vi "Save.vi"(8 "error in (no error)":errorcluster, 10 "Resampling Array":i32[](array[numeric]), 11 "DAQ Class in":refnum<class "DAQ Class.lvclass">) -> (0 "error out":errorcluster, 3 "DAQ Class out":refnum<class "DAQ Class.lvclass">)   [LabVIEW 2014, in "DAQ Class.lvclass"]
uses:
  DAQ Class.lvclass
  DAQ Class.lvclass/DAQ Class.ctl
  <vilib>/Utility/config.llb/Write Key (Double).vi
  <vilib>/Utility/config.llb/Write Key (I32).vi
  <vilib>/Utility/config.llb/Write Key (U32).vi
  <vilib>/Utility/config.llb/NI_LVConfig.lvlib
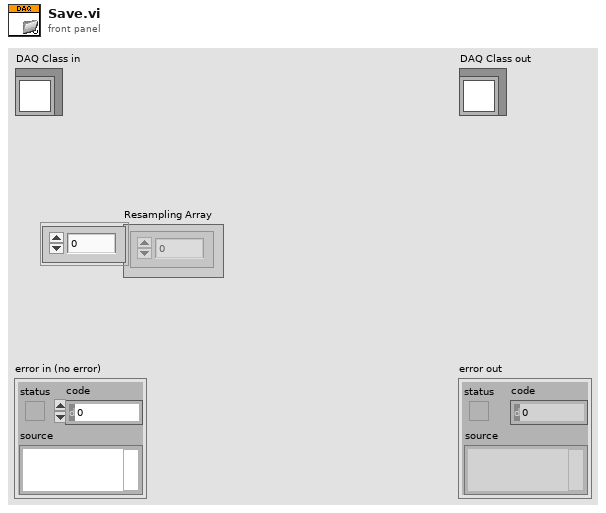
[diagram p1: front panel]
types:
  T1 = typedef "DAQ Class.lvclass/DAQ Parameters.ctl" = cluster{"Points Per A-Scan":u32, "A-Scans Per B-Scan":u32, "Number of B-Scans":u32, "A-Scans Per Transfer":u32, "Trigger Voltage":sgl, "Trigger Source":T2, "Trigger Slope":T3, "Channel":T4, "Clock":T5, "Bits per Sample":dbl, "Range":dbl}
  T2 = typedef "DAQ Class.lvclass/Trigger Source.ctl" = enum16{"External", "Channel A", "Channel B"}
  T3 = typedef "DAQ Class.lvclass/Trigger Slope.ctl" = enum16{"Rising", "Falling"}
  T4 = typedef "OCT DAQ Channel Data Type.ctl" = enum16{"Channel 1", "Channel 2", "Channel 1 and 2"}
  T5 = typedef "DAQ Class.lvclass/Clock Control.ctl" = enum16{"Internal Clock", "External Clock"}
  T6 = typedef "NI_LVConfig.lvlib/Config Data RefNum.ctl" = refnum<k1>
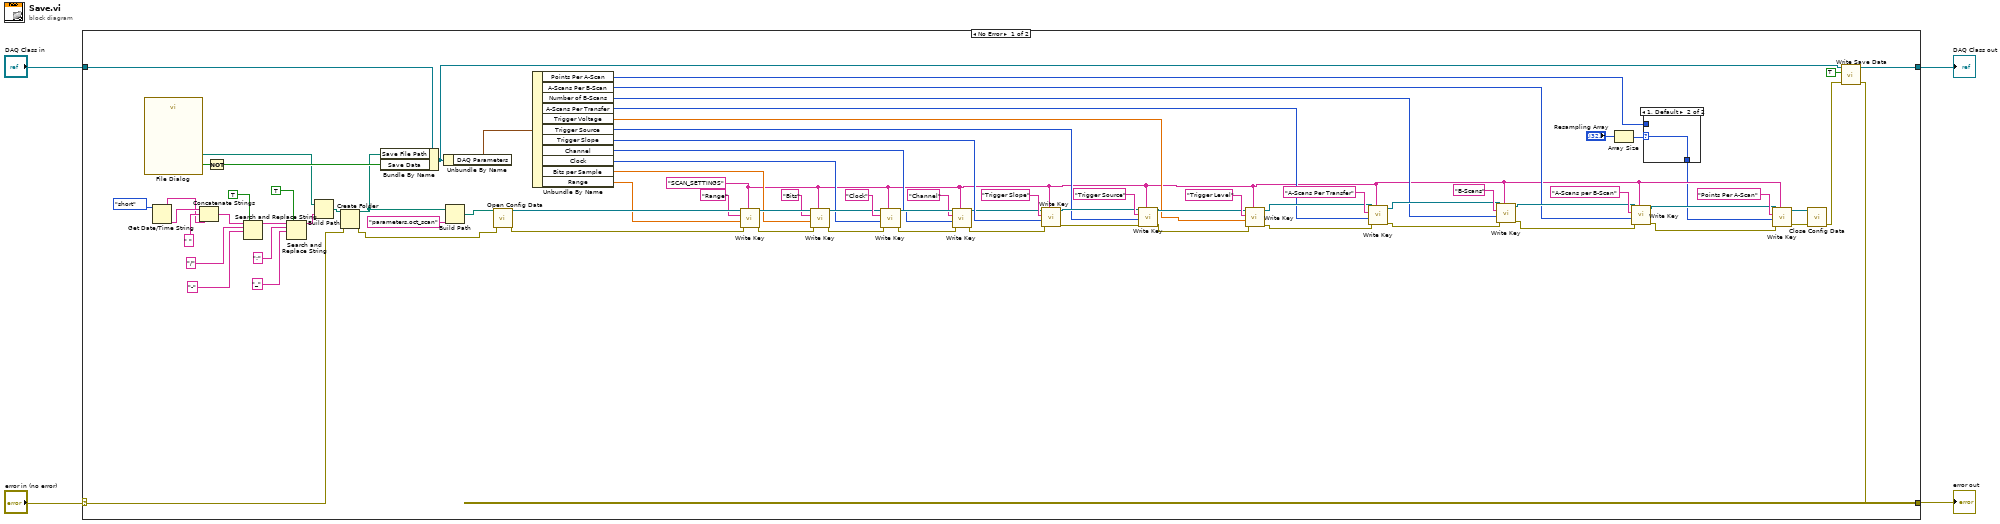
[diagram p0: block diagram]
diagram:
  n1 = case shown="No Error" "error in (no error)" {
    selector: "error in (no error)" -> [w66 w87]
    tunnel: [w8 w87] -> w3
    tunnel: [w7 w86] -> w1
    tunnel: "DAQ Class in" -> [w56 w86]
    frame No Error {
      w17 = "SCAN_SETTINGS" ("section")
      n2 = call "File Dialog"() -> ("selected path"=w77:path, "cancelled"=w83:bool)  [unwired: 12 in, 2 out]
      n3 = Get Date/Time String(date format (0)=enum16{"short", "long", "abbreviated"}."short") -> (date string=w79:string, time string=w80:string)  [unwired: 2 in]
      n4 = Concatenate Strings(w80, " " ("string"), w79) -> (w75:string)
      n5 = Not(x=w83) -> (.not. x?=w82:bool)
      n6 = Search and Replace String(replace all?=TRUE ("replace all? (F)"), input string=w75, search string="/", replace string="-" ("search string")) -> (result string=w72:string)  [unwired: 4 in, 3 out]
      n7 = Search and Replace String(replace all?=TRUE ("replace all? (F)"), input string=w72, search string=":", replace string="_" ("search string")) -> (result string=w71:string)  [unwired: 4 in, 3 out]
      n8 = Build Path(base path=w77, name or relative path=w71) -> (appended path=w67:path)
      n9 = Create Folder(path (use dialog)=w67, error in=w66) -> (created path=w65:path, error out=w62:errorcluster)  [unwired: 1 in, 1 out]
      n10 = Bundle By Name(cluster=w56, "Save File Path"=w65, "Save Data"=w82) -> (w5:refnum<class "DAQ Class.lvclass">)
      n11 = Unbundle By Name(w5) -> ("DAQ Parameters"=w59:T1)
      n12 = Build Path(base path=w65, name or relative path="parameters.oct_scan") -> (appended path=w63:path)
      n13 = call <vilib>:"Open Config Data.vi"("error in (no error)"=w62, "configuration file path"=w63) -> ("error out"=w60:errorcluster, "refnum"=w61:T6)  [unwired: 7 in, 1 out]
      n14 = Unbundle By Name(w59) -> ("Points Per A-Scan"=w11:u32, "A-Scans Per B-Scan"=w21:u32, "Number of B-Scans"=w25:u32, "A-Scans Per Transfer"=w29:u32, "Trigger Voltage"=w33:sgl, "Trigger Source"=w37:T2, "Trigger Slope"=w42:T3, "Channel"=w45:T4, "Clock"=w49:T5, "Bits per Sample"=w53:dbl, "Range"=w58:dbl)
      n15 = call-poly <vilib>:"Write Key.vi"("section"=w17, "error in (no error)"=w60, "value"=w58, "key"="Range", "refnum"=w61) -> ("error out"=w14:errorcluster, "refnum out"=w55:T6)  [unwired: 4 in, 1 out]
      n16 = call-poly <vilib>:"Write Key.vi"("section"=w17, "error in (no error)"=w14, "value"=w53, "key"="Bits", "refnum"=w55) -> ("error out"=w51:errorcluster, "refnum out"=w50:T6)  [unwired: 4 in, 1 out]
      n17 = call-poly <vilib>:"Write Key.vi"("section"=w17, "error in (no error)"=w51, "value"=w49, "key"="Clock", "refnum"=w50) -> ("error out"=w47:errorcluster, "refnum out"=w48:T6)  [unwired: 4 in, 1 out]
      n18 = call-poly <vilib>:"Write Key.vi"("section"=w17, "error in (no error)"=w47, "value"=w45, "key"="Channel", "refnum"=w48) -> ("error out"=w43:errorcluster, "refnum out"=w41:T6)  [unwired: 4 in, 1 out]
      n19 = call-poly <vilib>:"Write Key.vi"("section"=w17, "error in (no error)"=w43, "value"=w42, "key"="Trigger Slope", "refnum"=w41) -> ("error out"=w39:errorcluster, "refnum out"=w38:T6)  [unwired: 4 in, 1 out]
      n20 = call-poly <vilib>:"Write Key.vi"("section"=w17, "error in (no error)"=w39, "value"=w37, "key"="Trigger Source", "refnum"=w38) -> ("error out"=w35:errorcluster, "refnum out"=w34:T6)  [unwired: 4 in, 1 out]
      n21 = call-poly <vilib>:"Write Key.vi"("section"=w17, "error in (no error)"=w35, "value"=w33, "key"="Trigger Level", "refnum"=w34) -> ("error out"=w31:errorcluster, "refnum out"=w30:T6)  [unwired: 4 in, 1 out]
      n22 = call-poly <vilib>:"Write Key.vi"("section"=w17, "error in (no error)"=w31, "value"=w29, "key"="A-Scans Per Transfer", "refnum"=w30) -> ("error out"=w27:errorcluster, "refnum out"=w26:T6)  [unwired: 4 in, 1 out]
      n23 = call-poly <vilib>:"Write Key.vi"("section"=w17, "error in (no error)"=w27, "value"=w25, "key"="B-Scans", "refnum"=w26) -> ("error out"=w22:errorcluster, "refnum out"=w23:T6)  [unwired: 4 in, 1 out]
      n24 = Array Size(array="Resampling Array") -> (size(s)=w12:i32)
      n25 = call-poly <vilib>:"Write Key.vi"("section"=w17, "error in (no error)"=w22, "value"=w21, "key"="A-Scans per B-Scan", "refnum"=w23) -> ("error out"=w18:errorcluster, "refnum out"=w19:T6)  [unwired: 4 in, 1 out]
      n26 = case shown="1, Default" w12 {
        selector: w12 -> [_ w85]
        tunnel: w11 -> [w84 _]
        tunnel: [w84 w85] -> w10
        frame 0 {
        }
        frame 1, Default {
        }
      }
      n27 = call-poly <vilib>:"Write Key.vi"("section"=w17, "error in (no error)"=w18, "value"=w10, "key"="Points Per A-Scan", "refnum"=w19) -> ("error out"=w16:errorcluster, "refnum out"=w15:T6)  [unwired: 4 in, 1 out]
      n28 = call <vilib>:"Close Config Data.vi"("error in (no error)"=w16, "refnum"=w15) -> ("error out"=w9:errorcluster)  [unwired: 8 in, 1 out]
      n29 = call-dynamic "Write Save Data.vi"("error in (no error)"=w9, "Save Data"=TRUE, "DAQ Class in"=w5) -> ("error out"=w8:errorcluster, "DAQ Class out"=w7:refnum<class "DAQ Class.lvclass">)  [unwired: 7 in]
    }
    frame Error {
    }
  }
  "error out" <- w3
  "DAQ Class out" <- w1
